vi "SteptoRun.vi"(8 "error in (no error)":errorcluster, 10 "StepSetup":string, 11 "StepData.lvclass In":refnum<class "StepData.lvclass">) -> (0 "error out":errorcluster, 2 "StepDataArray":refnum<class "StepData.lvclass">[](array[class]))   [LabVIEW 2014, in "Project.lvclass"]
uses:
  Project.lvclass
  StepData/StepData.lvclass
  StepSetupDataTypeDefine.ctl
  StepData/Control/AllStepTypeData.ctl
  StepData/Control/StepTypeEnum.ctl
  StepData/Control/MoveData.ctl
  StepData/Control/MeasureData.ctl
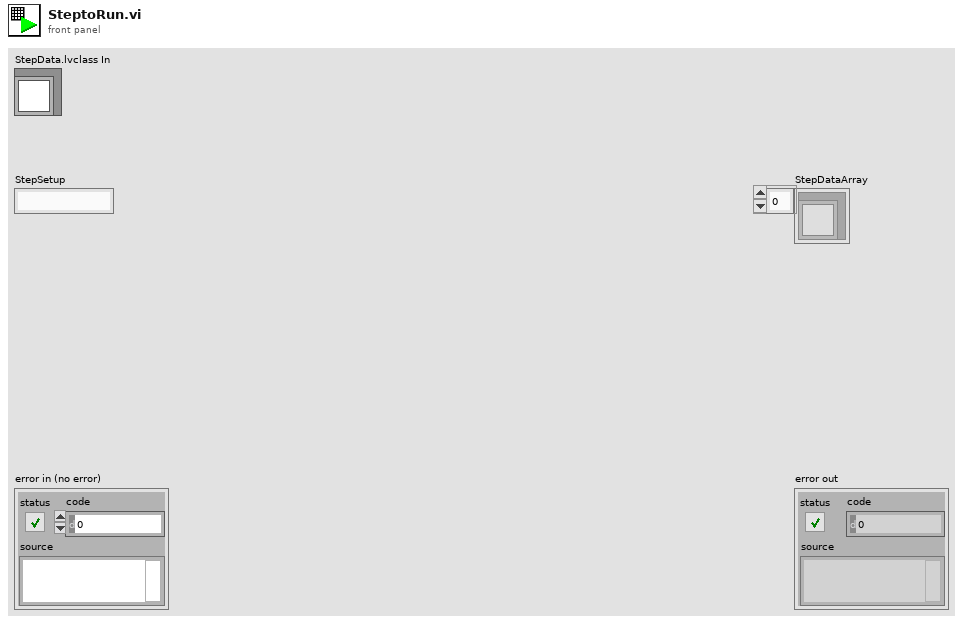
[diagram p1: front panel]
types:
  T1 = typedef "Project.lvclass/StepSetupDataTypeDefine.ctl" = cluster{"AllStepTypeData":T2}[]
  T2 = typedef "StepData.lvclass/AllStepTypeData.ctl" = cluster{"StepName":string, "StepTypeEnum":T3, "MoveData":T4, "MeasureData":T5}
  T3 = typedef "StepData.lvclass/StepTypeEnum.ctl" = enum16{"Move", "Measure"}
  T4 = typedef "StepData.lvclass/MoveData.ctl" = cluster{"Axis":u16, "Position":dbl, "Speed":dbl, "Acc/Dec":dbl, "Mode":u16}
  T5 = typedef "StepData.lvclass/MeasureData.ctl" = cluster{"Sensor No.":i32, "Log?":bool}
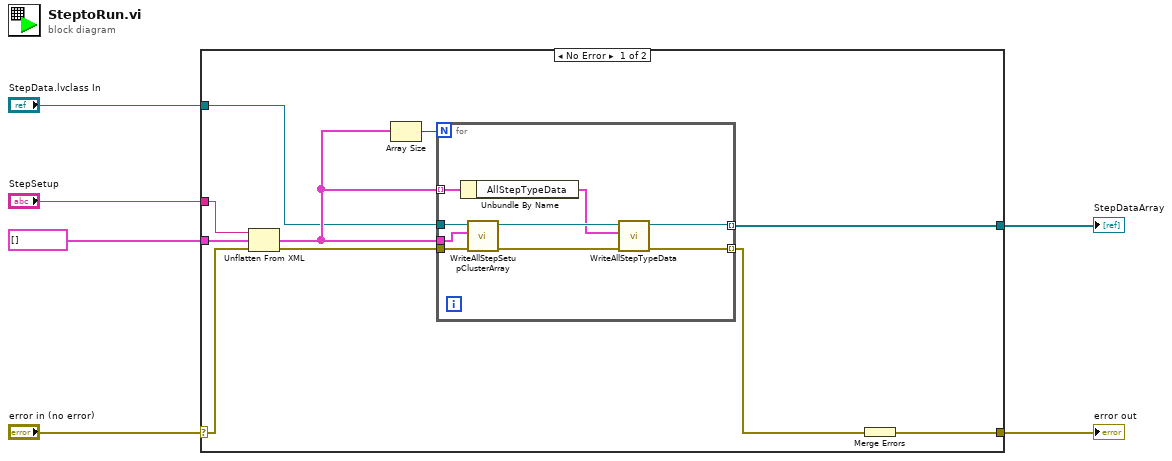
[diagram p0: block diagram]
diagram:
  n1 = case shown="No Error" "error in (no error)" {
    selector: "error in (no error)" -> [w15 w26]
    tunnel: [w10 w26] -> w5
    tunnel: T1 [] ("StepSetupClusterArray") -> [w16 _]
    tunnel: [w9 _] -> w3
    tunnel: "StepSetup" -> [w8 _]
    tunnel: "StepData.lvclass In" -> [w7 _]
    frame No Error {
      n2 = Unflatten From XML(xml string=w8, type=w16, error in (no error)=w15) -> (value=w12:T1, error out=w14:errorcluster)
      n3 = Array Size(array=w12) -> (size(s)=w13:i32)
      n4 = for {
        N: w13 -> [_]
        tunnel: w12 -> [w24] mode=indexing
        tunnel: w14 -> [w25]
        tunnel: w12 -> [w23]
        tunnel: [w19] -> w9 mode=indexing
        tunnel: [w18] -> w11 mode=indexing
        tunnel: w7 -> [w17]
        n5 = Unbundle By Name(w24) -> ("AllStepTypeData"=w20:T2)
        n6 = call "WriteAllStepSetupClusterArray.vi"("error in (no error)"=w25, "AllStepSetupClusterArray"=w23, "StepData.lvclass In"=w17) -> ("error out"=w22:errorcluster, "StepData.lvclass Out"=w21:refnum<class "StepData.lvclass">)  [unwired: 7 in]
        n7 = call "WriteAllStepTypeData.vi"("error in (no error)"=w22, "AllStepTypeData"=w20, "StepData.lvclass In"=w21) -> ("error out"=w18:errorcluster, "StepData.lvclass Out"=w19:refnum<class "StepData.lvclass">)  [unwired: 7 in]
      }
      n8 = Merge Errors(w11) -> (w10:errorcluster)
    }
    frame Error {
    }
  }
  "error out" <- w5
  "StepDataArray" <- w3
